vi "_Main.vi"() -> ()   [LabVIEW 2017]
uses:
  Controls/RegisterValue.ctl
panel:
  in  "Frame rate":T1
  in  "int. Time":T1
  in  "stop":bool
  in  "remote port or service name":u16
  in  "IP Address":string
  # "ToF System"
  # "e"
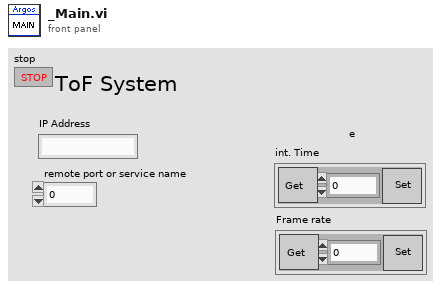
[diagram p1: front panel]
types:
  T1 = typedef "RegisterValue.ctl" = cluster{"Value":dbl, "Set":bool, "Get 2":bool}
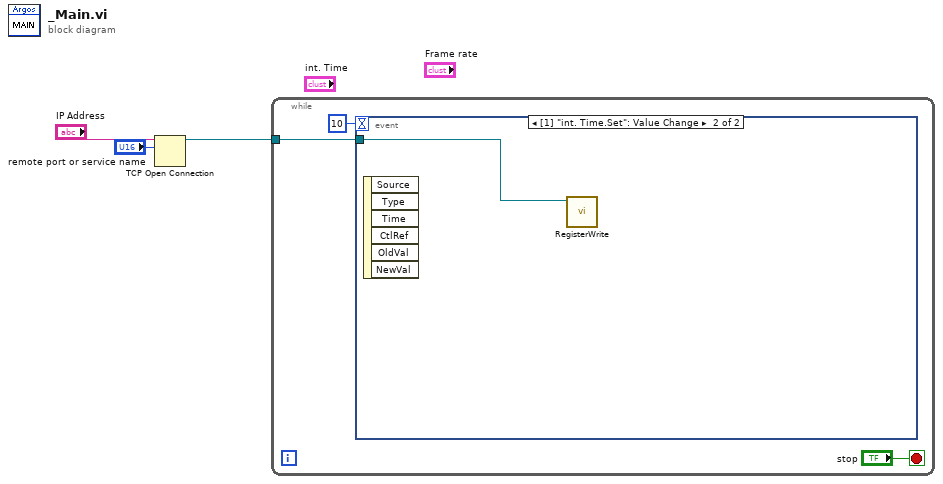
[diagram p0: block diagram]
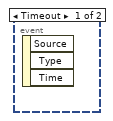
[diagram p2: hidden frame]
diagram:
  n1 = TCP Open Connection(address="IP Address", remote port or service name="remote port or service name") -> (connection ID=w1:refnum<k5>)  [unwired: 3 in, 1 out]
  n2 = while {
    tunnel: w1 -> [w4]
    stop <- "stop" stop-if-true
    n3 = event shown="[1] \"int. Time.Set\": Value Change" {
      selector: _ -> [_ _]
      dyn-events: _ -> [_ _]
      timeout: 10 -> [_ _]
      tunnel: w4 -> [_ w7]
      event Timeout {
        n4 = event-data() -> ()  [unwired: 1 in, 3 out]
      }
      event Value Change {
        n5 = event-data() -> ()  [unwired: 1 in, 6 out]
        n6 = call "RegisterWrite.vi"("connection ID In"=w7) -> ()  [unwired: 9 in, 2 out]
      }
    }
  }
